vi "storage.writer.vi"(7 "Data Source RID":string, 8 "error in":errorcluster, 9 "Points":T1(array[cluster]), 10 "Channel":string, 11 "Nominal Client in":refnum<class "Nominal Client.lvclass">) -> (0 "error out":errorcluster, 2 "Response body":string, 3 "Nominal Client out":refnum<class "Nominal Client.lvclass">, 4 "Response Headers":refnum<class "Response Headers.lvclass">)   [LabVIEW 2020, in "Nominal Client.lvclass"]
uses:
  Nominal Client.lvclass
  Nominal Client.lvclass/Nominal Client.ctl
  <vilib>/addons/_JKI.lib/REST Client/classes/Response Headers/Response Headers.lvclass
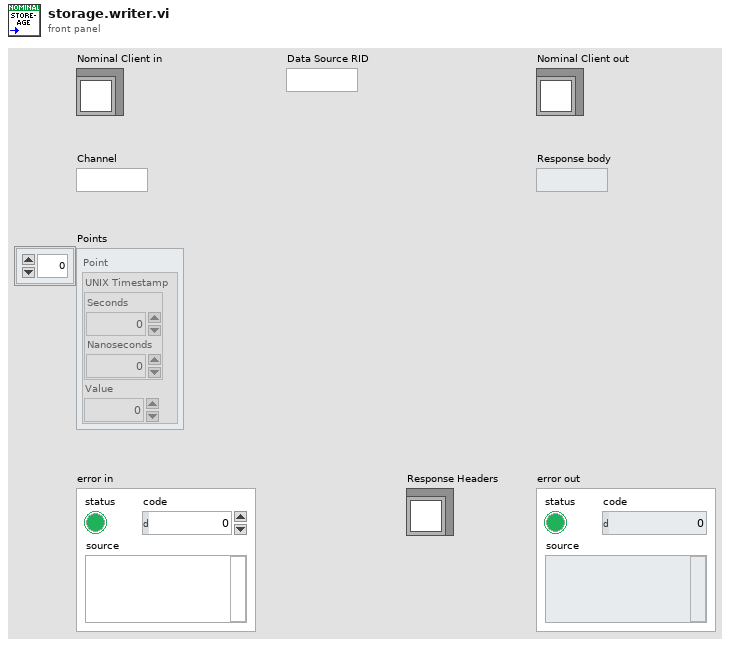
[diagram p1: front panel]
types:
  T1 = cluster{"UNIX Timestamp":cluster{"Seconds":i64, "Nanoseconds":i64}, "Value":dbl}[]
  T2 = cluster{"batches":cluster{"channel":string, "points":cluster{"type":string, "double":cluster{"timestamp":cluster{"nanos":i32, "seconds":i32}, "value":dbl}[]}}[], "dataSourceRid":string}
  T3 = cluster{"type":string, "Points":cluster{"UNIX Timestamp":cluster{"Seconds":i64, "Nanoseconds":i64}, "Value":dbl}[]}
  T4 = cluster{"Channel":string, cluster{"type":string, "Points":cluster{"UNIX Timestamp":cluster{"Seconds":i64, "Nanoseconds":i64}, "Value":dbl}[]}}
  T5 = cluster{"Channel":string, cluster{"type":string, "Points":cluster{"UNIX Timestamp":cluster{"Seconds":i64, "Nanoseconds":i64}, "Value":dbl}[]}}[]
  T6 = cluster{cluster{"Channel":string, cluster{"type":string, "Points":cluster{"UNIX Timestamp":cluster{"Seconds":i64, "Nanoseconds":i64}, "Value":dbl}[]}}[], "Data Source RID":string}
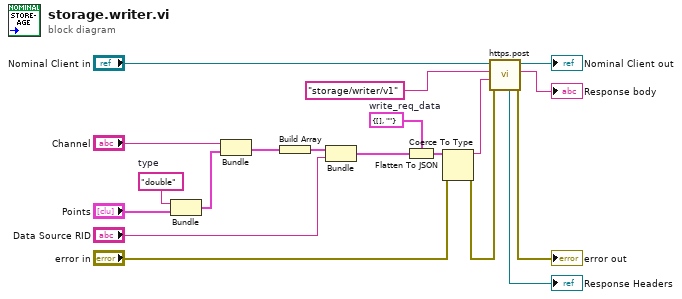
[diagram p0: block diagram]
diagram:
  w5 = T2 {"batches"=[], "dataSourceRid"=""}  # write_req_data
  w13 = "double"  # type
  n1 = Bundle("type"=w13, "Points"="Points") -> (w11:T3)  [unwired: 1 in]
  n2 = Bundle("Channel"="Channel", w11) -> (w9:T4)  [unwired: 1 in]
  n3 = Build Array(w9) -> (w8:T5)
  n4 = Bundle(w8, "Data Source RID"="Data Source RID") -> (w6:T6)  [unwired: 1 in]
  n5 = Coerce To Type(0:w6, 1:w5) -> (2:w4:T2)
  n6 = Flatten To JSON(anything=w4, error in (no error)="error in") -> (JSON string=w1:string, 11:w2:errorcluster)  [unwired: 1 in]
  n7 = call "https.post.vi"("error in"=w2, "Request body"=w1, "Path"="storage/writer/v1", "Nominal Client in"="Nominal Client in") -> ("error out"=→"error out":errorcluster, "Response"=→"Response body":string, "Nominal Client out"=→"Nominal Client out":refnum<class "Nominal Client.lvclass">, "Response Headers"=→"Response Headers":refnum<class "Response Headers.lvclass">)  [unwired: 4 in]
